vi "GetAnalyzerParameterInfo.vi"(8 "error in":errorcluster, 10 "Parameter Name":string, 11 "connection ID in":refnum<k5>) -> (0 "error out":errorcluster, 1 "Error Info":T1, 2 "Parameter Info":T2, 3 "connection ID out":refnum<k5>, 4 "Log String":string, 5 "OK":bool)   [LabVIEW 2020, in "ProdigyRemoteControl.lvlib"]
uses:
  ProdigyRemoteControl.lvlib
  DEFINITIONS/DEF_AnalyzerParaInfo.ctl
  DEFINITIONS/DEF_RcError.ctl
  DEFINITIONS/DEF_RcCmd.ctl
  <vilib>/regexp/Match Regular Expression.xnode
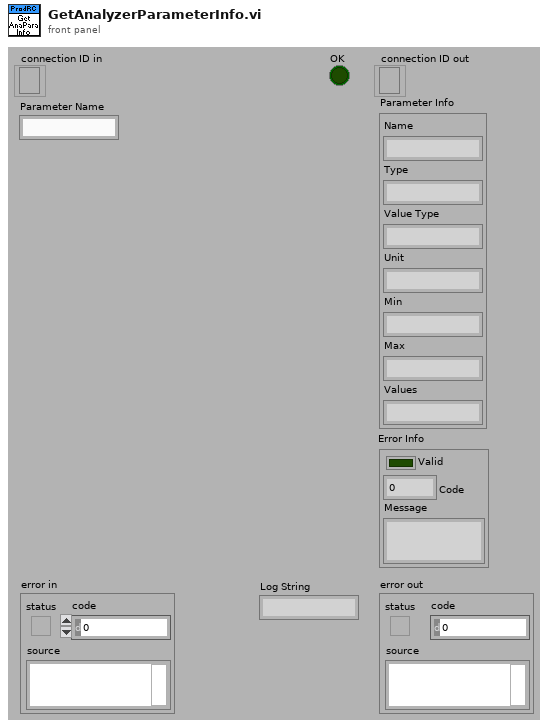
[diagram p1: front panel]
types:
  T1 = typedef "ProdigyRemoteControl.lvlib/DEF_RcError.ctl" = cluster{"Valid":bool, "Code":u16, "Message":string}
  T2 = typedef "ProdigyRemoteControl.lvlib/DEF_AnalyzerParaInfo.ctl" = cluster{"Name":string, "Type":string, "Value Type":string, "Unit":string, "Min":string, "Max":string, "Values":string}
  T3 = typedef "ProdigyRemoteControl.lvlib/DEF_RcCmd.ctl" = string
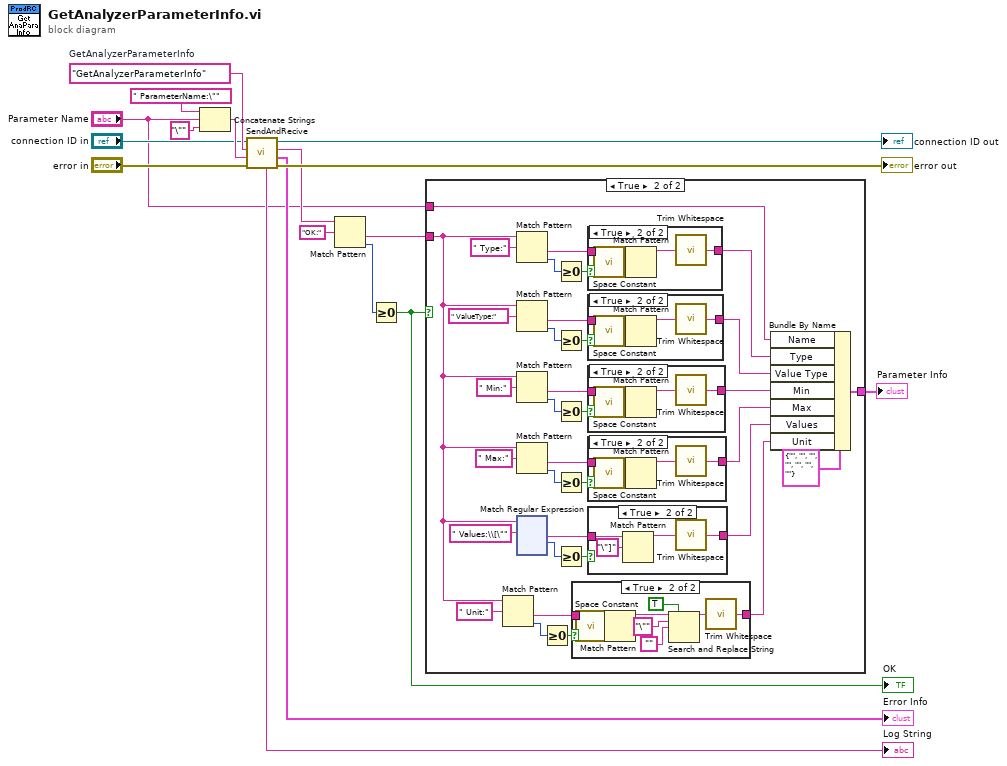
[diagram p0: block diagram]
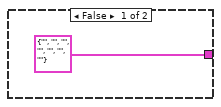
[diagram p2: hidden frame]
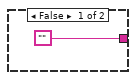
[diagram p3: hidden frame]
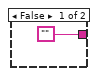
[diagram p4: hidden frame]
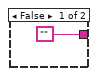
[diagram p5: hidden frame]
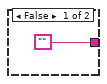
[diagram p6: hidden frame]
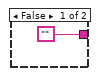
[diagram p7: hidden frame]
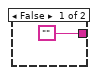
[diagram p8: hidden frame]
diagram:
  w17 = T3 "GetAnalyzerParameterInfo"  # GetAnalyzerParameterInfo
  n1 = Concatenate Strings(" ParameterName:\"", "Parameter Name", "\"" ("string")) -> (w16:string)
  n2 = call "SendAndRecive.vi"("error in"="error in", "Parameters"=w16, "Command"=w17, "connection ID in"="connection ID in") -> ("error out"=→"error out":errorcluster, "Error Info"=→"Error Info":T1, "Answer"=w7:string, "connection ID out"=→"connection ID out":refnum<k5>, "Log String"=→"Log String":string)  [unwired: 3 in]
  n3 = Match Pattern(string=w7, regular expression="OK:") -> (after substring=w3:string, offset past match=w5:i32)  [unwired: 1 in, 2 out]
  n4 = Greater Or Equal To 0?(x=w5) -> (x >= 0?=w4:bool)
  "OK" <- w4
  n5 = case shown="True" w4 {
    tunnel: w3 -> [_ w21]
    tunnel: "Parameter Name" -> [_ w30]
    tunnel: [T2 {"Name"="", "Type"="", "Value Type"="", "Unit"="", "Min"="", "Max"="", "Values"=""} ("DEF_ParameterInfo") w24] -> w1
    frame False {
    }
    frame True {
      n6 = Match Pattern(string=w21, regular expression=" Unit:") -> (after substring=w43:string, offset past match=w44:i32)  [unwired: 1 in, 2 out]
      n7 = Match Pattern(string=w21, regular expression=" Type:") -> (after substring=w49:string, offset past match=w51:i32)  [unwired: 1 in, 2 out]
      n8 = Match Pattern(string=w21, regular expression=" ValueType:") -> (after substring=w46:string, offset past match=w45:i32)  [unwired: 1 in, 2 out]
      n9 = Match Pattern(string=w21, regular expression=" Min:") -> (after substring=w38:string, offset past match=w37:i32)  [unwired: 1 in, 2 out]
      n10 = Match Pattern(string=w21, regular expression=" Max:") -> (after substring=w35:string, offset past match=w36:i32)  [unwired: 1 in, 2 out]
      n11 = xnode "Match Regular Expression"("input string"=w21, "regular expression"=" Values:\\[\"") -> ("after match"=w20:string, "offset past match"=w19:i32)  [unwired: 4 in, 3 out]
      n12 = Greater Or Equal To 0?(x=w44) -> (x >= 0?=w41:bool)
      n13 = Greater Or Equal To 0?(x=w51) -> (x >= 0?=w50:bool)
      n14 = Greater Or Equal To 0?(x=w45) -> (x >= 0?=w48:bool)
      n15 = Greater Or Equal To 0?(x=w37) -> (x >= 0?=w40:bool)
      n16 = Greater Or Equal To 0?(x=w36) -> (x >= 0?=w33:bool)
      n17 = Greater Or Equal To 0?(x=w19) -> (x >= 0?=w32:bool)
      n18 = case shown="True" w41 {
        tunnel: w43 -> [_ w187]
        tunnel: ["" w180] -> w23
        frame False {
        }
        frame True {
          n19 = call <vilib>:"Space Constant.vi"() -> ("String"=w186:string)
          n20 = Match Pattern(string=w187, regular expression=w186) -> (before substring=w184:string)  [unwired: 1 in, 3 out]
          n21 = Search and Replace String(replace all?=TRUE ("replace all? (F)"), input string=w184, search string="\"", replace string="") -> (result string=w185:string)  [unwired: 4 in, 3 out]
          n22 = call <vilib>:"Trim Whitespace.vi"("string"=w185) -> ("trimmed string"=w180:string)  [unwired: 1 in]
        }
      }
      n23 = case shown="True" w50 {
        tunnel: w49 -> [_ w197]
        tunnel: ["" w195] -> w29
        frame False {
        }
        frame True {
          n24 = call <vilib>:"Space Constant.vi"() -> ("String"=w196:string)
          n25 = Match Pattern(string=w197, regular expression=w196) -> (before substring=w194:string)  [unwired: 1 in, 3 out]
          n26 = call <vilib>:"Trim Whitespace.vi"("string"=w194) -> ("trimmed string"=w195:string)  [unwired: 1 in]
        }
      }
      n27 = case shown="True" w48 {
        tunnel: w46 -> [_ w192]
        tunnel: ["" w190] -> w28
        frame False {
        }
        frame True {
          n28 = call <vilib>:"Space Constant.vi"() -> ("String"=w191:string)
          n29 = Match Pattern(string=w192, regular expression=w191) -> (before substring=w189:string)  [unwired: 1 in, 3 out]
          n30 = call <vilib>:"Trim Whitespace.vi"("string"=w189) -> ("trimmed string"=w190:string)  [unwired: 1 in]
        }
      }
      n31 = case shown="True" w40 {
        tunnel: w38 -> [_ w178]
        tunnel: ["" w176] -> w27
        frame False {
        }
        frame True {
          n32 = call <vilib>:"Space Constant.vi"() -> ("String"=w177:string)
          n33 = Match Pattern(string=w178, regular expression=w177) -> (before substring=w175:string)  [unwired: 1 in, 3 out]
          n34 = call <vilib>:"Trim Whitespace.vi"("string"=w175) -> ("trimmed string"=w176:string)  [unwired: 1 in]
        }
      }
      n35 = case shown="True" w33 {
        tunnel: w35 -> [_ w173]
        tunnel: ["" w171] -> w26
        frame False {
        }
        frame True {
          n36 = call <vilib>:"Space Constant.vi"() -> ("String"=w172:string)
          n37 = Match Pattern(string=w173, regular expression=w172) -> (before substring=w170:string)  [unwired: 1 in, 3 out]
          n38 = call <vilib>:"Trim Whitespace.vi"("string"=w170) -> ("trimmed string"=w171:string)  [unwired: 1 in]
        }
      }
      n39 = case shown="True" w32 {
        tunnel: w20 -> [_ w168]
        tunnel: ["" w166] -> w25
        frame False {
        }
        frame True {
          n40 = Match Pattern(string=w168, regular expression="\"]") -> (before substring=w165:string)  [unwired: 1 in, 3 out]
          n41 = call <vilib>:"Trim Whitespace.vi"("string"=w165) -> ("trimmed string"=w166:string)  [unwired: 1 in]
        }
      }
      n42 = Bundle By Name(cluster=T2 {"Name"="", "Type"="", "Value Type"="", "Unit"="", "Min"="", "Max"="", "Values"=""} ("DEF_ParameterInfo"), "Name"=w30, "Type"=w29, "Value Type"=w28, "Min"=w27, "Max"=w26, "Values"=w25, "Unit"=w23) -> (w24:T2)
    }
  }
  "Parameter Info" <- w1
